vi "Phasics raw array to image.vi"(8 "error in (no error)":errorcluster, 11 "Phasics Camera in":refnum<class "Phasics Camera.lvclass">) -> (0 "error out":errorcluster, 1 "Image out":i16[][](array[numeric]), 3 "Phasics Camera out":refnum<class "Phasics Camera.lvclass">, 4 "String out":string)   [LabVIEW 2013, in "Phasics Camera.lvclass"]
uses:
  Phasics Camera.lvclass
  Phasics Camera.lvclass/Phasics Camera.ctl
  CompressAndUpdate(IMAQ Image).vi
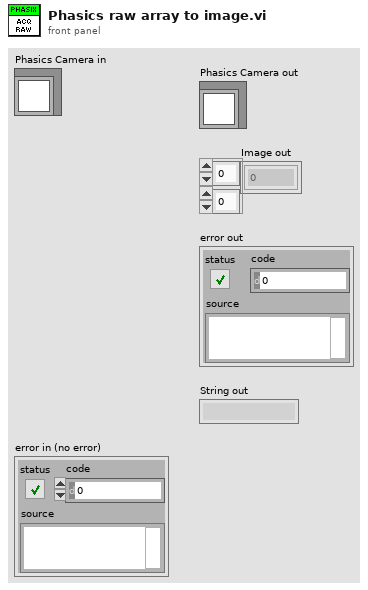
[diagram p1: front panel]
types:
  T1 = typedef "OnOffTypeDef.ctl" = enum16{"off", "on"}
  T2 = typedef "IMAQ Image.ctl" = refnum<image>
  T3 = typedef "Refnum SDKSID4 session.ctl" = refnum<k1>
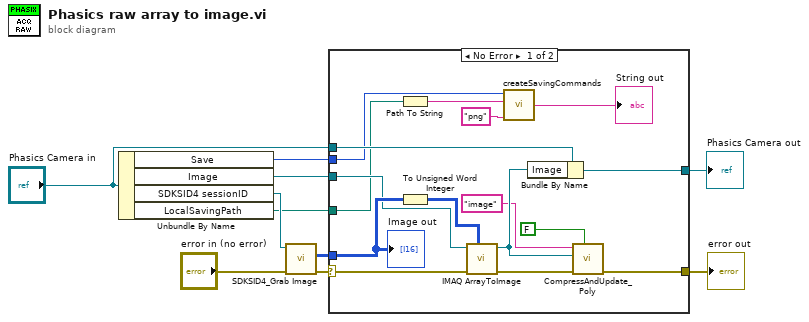
[diagram p0: block diagram]
diagram:
  n1 = Unbundle By Name("Phasics Camera in") -> ("Save"=w2:T1, "Image"=w3:T2, "SDKSID4 sessionID"=w4:T3, "LocalSavingPath"=w1:path)
  n2 = call "SDKSID4_Grab Image.vi"("error in (no error)"="error in (no error)", "SDKSID4 session In"=w4) -> ("error out"=w6:errorcluster, "Image"=w8:i16[][])  [unwired: 6 in, 1 out]
  n3 = case shown="No Error" w6 {
    selector: w6 -> [w17 w27]
    tunnel: [w25 w28] -> w10
    tunnel: "Phasics Camera in" -> [w24 w28]
    tunnel: w8 -> [w22 _]
    tunnel: [w15 w27] -> w7
    tunnel: w3 -> [w14 _]
    tunnel: w2 -> [w13 _]
    tunnel: w1 -> [w12 _]
    frame No Error {
      n4 = Path To String(path=w12) -> (string=w11:string)
      n5 = To Unsigned Word Integer(number=w22) -> (unsigned 16bit integer=w23:u16[][])
      n6 = call "IMAQ ArrayToImage"("Image Pixels (U16)"=w23, "error in (no error)"=w17, "Image"=w14) -> ("error out"=w16:errorcluster, "Image Out"=w26:T2)  [unwired: 7 in]
      n7 = call "createSavingCommands.vi"("extension"="png" ("Fileextension"), "Saving Path (local)"=w11, "Save"=w13) -> ("String"=→"String out":string)  [unwired: 1 in]
      n8 = Bundle By Name(cluster=w24, "Image"=w26) -> (w25:refnum<class "Phasics Camera.lvclass">)
      n9 = call-poly "CompressAndUpdate_Poly.vi"("force CVT update (false)"=FALSE, "error in"=w16, "IMAQ Image"=w26, "command or variable name"="image") -> ("error out"=w15:errorcluster)  [unwired: 7 in]
      "Image out" <- w22
    }
    frame Error {
    }
  }
  "error out" <- w7
  "Phasics Camera out" <- w10
